vi "空调监测配置同步 (子VI).vi"(11 "Boolean输入":refnum<vi>) -> ()   [LabVIEW 2016, in "环境动力监测库.lvlib" / "空调库.lvlib"]
uses:
  <vilib>/Utility/config.llb/NI_LVConfig.lvlib
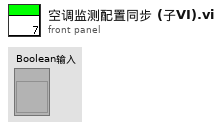
[diagram p1: front panel]
types:
  T1 = cluster{"分支":enum16{"open", "read", "write", "close"}, "字符串":string}
  T2 = cluster{"监测项描述:输出":string, "连接方式":enum16{"串口", "TCP"}, "端口":string, "IP address:":string, "Port:":string, "站号":u64, "传感器型号":string, "波特率":u64, "data bits":u64, "停止位":u16, "奇偶校验":u16}
  T3 = typedef "NI_LVConfig.lvlib/Config Data RefNum.ctl" = refnum<k1>
  T4 = cluster{"baud rate (bps)":u32, "stop bits":u16, "parity":u16, "flow control":u16, "timeout":u32, "retries":i32}
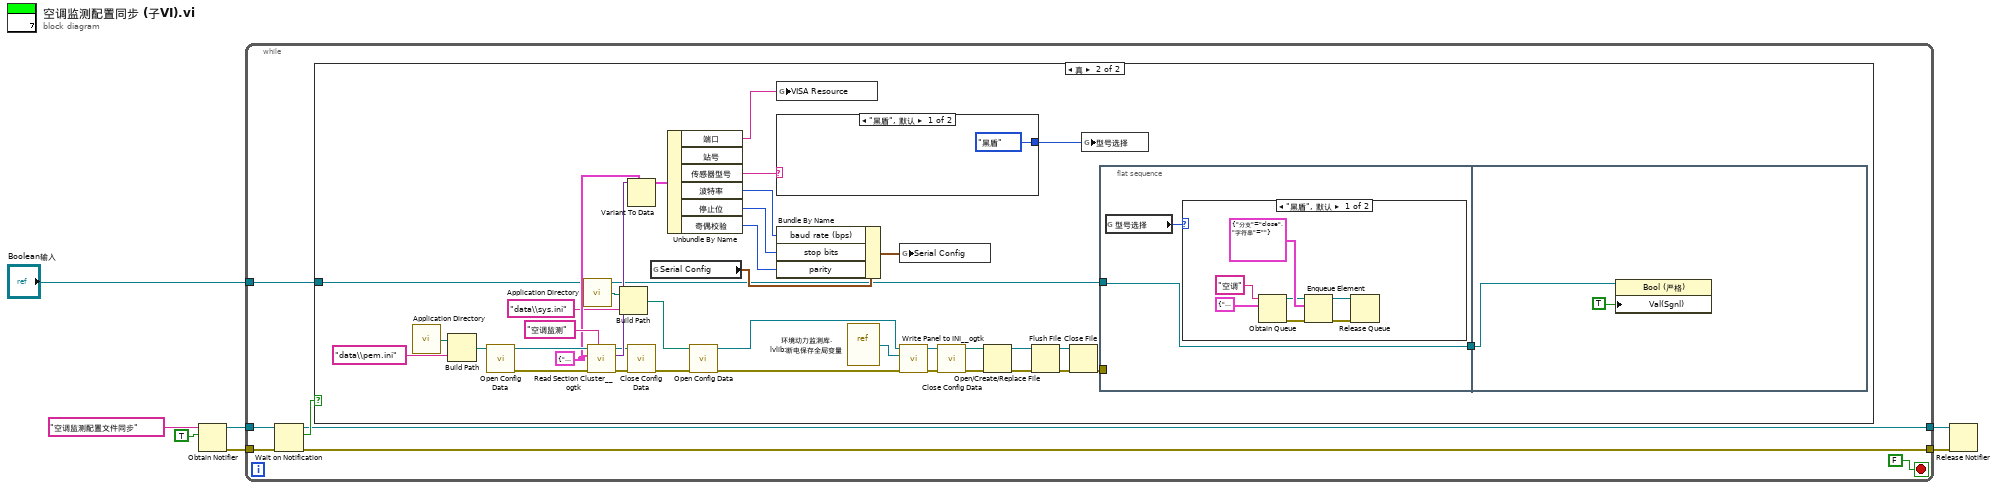
[diagram p0: block diagram]
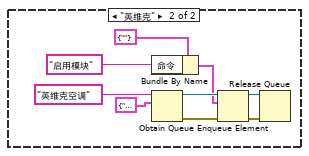
[diagram p3: hidden frame]
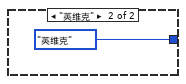
[diagram p4: hidden frame]
diagram:
  n1 = Obtain Notifier(name (unnamed)="空调监测配置文件同步" ("名称（未命名）"), notification data type=TRUE) -> (notifier out=w5:refnum<notifier>, error out=w4:errorcluster)  [unwired: 2 in, 1 out]
  n2 = while {
    tunnel: w5 -> [w14]
    tunnel: w4 -> [w13]
    tunnel: [w10] -> w3
    tunnel: [w9] -> w2
    tunnel: "Boolean输入" -> [w8]
    stop <- FALSE stop-if-true
    n3 = Wait on Notification(notifier=w14, error in (no error)=w13) -> (notifier out=w10:refnum<notifier>, notification=w12:bool, error out=w9:errorcluster)  [unwired: 2 in, 1 out]
    n4 = case shown="真" w12 {
      tunnel: w8 -> [_ w16]
      frame False {
      }
      frame True {
        w38 = T2 {"监测项描述:输出"="", "连接方式"=enum."串口", "端口"="", "IP address:"="", "Port:"="", "站号"=19200, "传感器型号"="", "波特率"=19200, "data bits"=8, "停止位"=10, "奇偶校验"=0} ("输入簇")
        n5 = call <vilib>:"Application Directory.vi"() -> ("Application Directory"=w42:path)
        n6 = Build Path(base path=w42, name or relative path="data\\pem.ini" ("名称或相对路径")) -> (appended path=w41:path)
        n7 = call <vilib>:"Open Config Data.vi"("configuration file path"=w41) -> ("error out"=w40:errorcluster, "refnum"=w39:T3)  [unwired: 8 in, 1 out]
        n8 = call <vilib>:"Application Directory.vi"() -> ("Application Directory"=w36:path)
        n9 = call <userlib>:"Read Section Cluster__ogtk.vi"("section (optional)"="空调监测", "error in (no error)"=w40, "Section Formatted Cluster Type"=w38, "refnum"=w39) -> ("error out"=w46:errorcluster, "Section Formatted Cluster"=w47:variant, "dup refnum"=w45:T3)  [unwired: 3 in, 2 out]
        n10 = Build Path(base path=w36, name or relative path="data\\sys.ini" ("名称或相对路径")) -> (appended path=w35:path)
        n11 = Variant To Data(type=w38, Variant=w47) -> (data=w48:T2)  [unwired: 1 in, 1 out]
        n12 = call <vilib>:"Close Config Data.vi"("error in (no error)"=w46, "refnum"=w45) -> ("error out"=w23:errorcluster)  [unwired: 8 in, 1 out]
        n13 = global read "断电保存全局变量.vi" "Serial Config"() -> (w19:T4)
        n14 = Unbundle By Name(w48) -> ("端口"=w21:string, "传感器型号"=w18:string, "波特率"=w49:u64, "停止位"=w50:u16, "奇偶校验"=w51:u16)  [unwired: 1 out]
        n15 = call <vilib>:"Open Config Data.vi"("error in (no error)"=w23, "configuration file path"=w35) -> ("error out"=w31:errorcluster, "refnum"=w34:T3)  [unwired: 7 in, 1 out]
        n16 = global write "断电保存全局变量.vi" "VISA Resource"(w21) -> ()
        n17 = case shown="\"黑盾\", 默认" w18 {
          tunnel: [enum16{"黑盾", "英维克"}."黑盾" ("型号选择") enum16{"黑盾", "英维克"}."英维克" ("型号选择")] -> w17
          frame "黑盾", Default {
          }
          frame "英维克" {
          }
        }
        n18 = Bundle By Name(cluster=w19, "baud rate (bps)"=w49, "stop bits"=w50, "parity"=w51) -> (w20:T4)
        n19 = vi-ref "环境动力监测库.lvlib:断电保存全局变量.vi"() -> (w33:refnum<vi>)
        n20 = global write "断电保存全局变量.vi" "Serial Config"(w20) -> ()
        n21 = call <userlib>:"Write Panel to INI__ogtk.vi"("error in (no error)"=w31, "VI ref"=w33, "refnum"=w34) -> ("error out"=w30:errorcluster, "refnum out"=w32:T3)  [unwired: 7 in]
        n22 = call <vilib>:"Close Config Data.vi"("error in (no error)"=w30, "refnum"=w32) -> ("error out"=w25:errorcluster, "file path"=w24:path)  [unwired: 8 in]
        n23 = Open/Create/Replace File(file path (use dialog)=w24, error in=w25) -> (refnum out=w28:refnum<file>, error out=w29:errorcluster)  [unwired: 4 in, 1 out]
        n24 = Flush File(refnum=w28, error in=w29) -> (refnum out=w27:refnum<file>, error out=w26:errorcluster)
        n25 = Close File(refnum=w27, error in=w26) -> (error out=w22:errorcluster)  [unwired: 1 out]
        n26 = global write "断电保存全局变量.vi" "型号选择"(w17) -> ()
        n27 = flat-sequence {
          tunnel: w22 -> [_]
          tunnel: w16 -> [w52]
          tunnel: [w52] -> w15
          tunnel: w15 -> [w70]
          frame #0 {
            n28 = global read "断电保存全局变量.vi" "型号选择"() -> (w53:enum16{"黑盾", "英维克"})
            n29 = case shown="\"黑盾\", 默认" w53 {
              frame "黑盾", Default {
                n30 = Obtain Queue(name (unnamed)="空调" ("名称（未命名）"), element data type=T1 {"分支"=enum."open", "字符串"="获取系统模拟量量化数据"}) -> (queue out=w57:refnum<queue>, error out=w56:errorcluster)  [unwired: 3 in, 1 out]
                n31 = Enqueue Element(queue=w57, element=T1 {"分支"=enum."close", "字符串"=""} ("元素"), error in (no error)=w56) -> (queue out=w55:refnum<queue>, error out=w54:errorcluster)  [unwired: 1 in, 1 out]
                n32 = Release Queue(queue=w55, error in (no error)=w54) -> ()  [unwired: 1 in, 3 out]
              }
              frame "英维克" {
                n33 = Bundle By Name(cluster=cluster{"命令":string} {"命令"=""} ("元素"), "命令"="启用模块" ("名称（未命名）")) -> (w65:cluster{"命令":string})
                n34 = Obtain Queue(name (unnamed)="英维克空调" ("名称（未命名）"), element data type=cluster{"命令":string} {"命令"="启用模块"} ("元素")) -> (queue out=w68:refnum<queue>, error out=w69:errorcluster)  [unwired: 3 in, 1 out]
                n35 = Enqueue Element(queue=w68, element=w65, error in (no error)=w69) -> (queue out=w62:refnum<queue>, error out=w61:errorcluster)  [unwired: 1 in, 1 out]
                n36 = Release Queue(queue=w62, error in (no error)=w61) -> ()  [unwired: 1 in, 3 out]
              }
            }
          }
          frame #1 {
            n37 = property on="属性节点" class="Bool (严格)"(reference=w70, "Val(Sgnl)"=TRUE) -> ()  [unwired: 1 in, 2 out]
          }
        }
      }
    }
  }
  n38 = Release Notifier(notifier=w3, error in (no error)=w2) -> ()  [unwired: 1 in, 3 out]
